vi "sv_Compute Next Time Offset at State.vi"(9 "time offset at previous state":dbl, 10 "duration of previous state":dbl, 11 "dt":dbl) -> (2 "time offset at next state":dbl)   [LabVIEW 2017, in "SoundVib_Generation.lvlib"]
uses:
  <vilib>/addons/_NISVFA/_Generation/SoundVib_Generation.lvlib
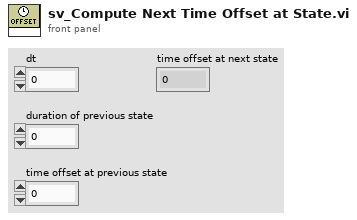
[diagram p1: front panel]
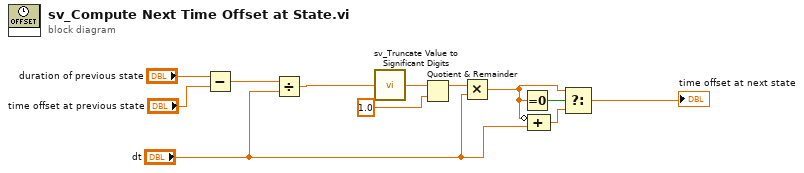
[diagram p0: block diagram]
diagram:
  n1 = Subtract(x="duration of previous state", y="time offset at previous state") -> (x-y=w7:dbl)
  n2 = Divide(x=w7, y="dt") -> (x/y=w6:dbl)
  n3 = call <vilib>:"sv_Truncate Value to Significant Digits.vi"("value"=w6) -> ("truncated value"=w5:dbl)  [unwired: 14 in]
  n4 = Quotient & Remainder(x=w5, y=1.0) -> (x-y*floor(x/y)=w3:dbl)  [unwired: 1 out]
  n5 = Multiply(x=w3, y="dt") -> (x*y=w1:dbl)
  n6 = Equal To 0?(x=w1) -> (x = 0?=w8:bool)
  n7 = Compound Arithmetic op=ADD(invert w1, "dt") -> (w9:dbl)
  n8 = Select(t=w1, s=w8, f=w9) -> (s? t:f=→"time offset at next state":dbl)
